vi "Delay.vi"(8 "error in (no error)":errorcluster, 9 "delay_value":u8=16 max=31 format="%1d", 10 "channel":u32, 11 "IP address":string="192.168.10.20") -> (0 "error out":errorcluster)   [LabVIEW 2017]
panel:
  in  "Read (TRUE)":bool
  out "Out":u8=16 format="%.0x"
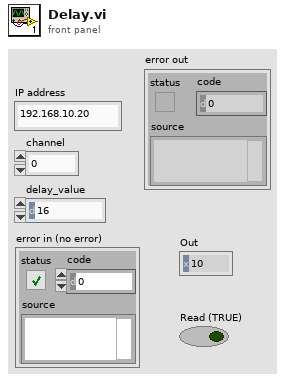
[diagram p1: front panel]
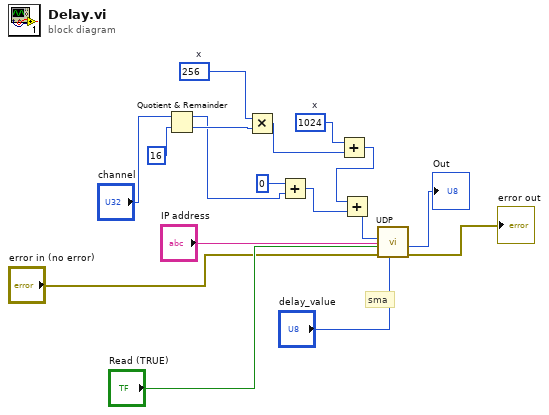
[diagram p0: block diagram]
diagram:
  w6 = u16 256  # x
  w4 = u16 1024  # x
  # "sma"
  n1 = Quotient & Remainder(x="channel", y=u32 16) -> (x-y*floor(x/y)=w1:u32, floor(x/y)=w5:u32)
  n2 = Multiply(x=w6, y=w5) -> (x*y=w3:u32)
  n3 = Add(x=u8 0, y=w1) -> (x+y=w11:u32)
  n4 = Add(x=w4, y=w3) -> (x+y=w2:u32)
  n5 = Add(x=w2, y=w11) -> (x+y=w15:u32)
  n6 = call "UDP.vi"("In"="delay_value", "error in (no error)"="error in (no error)", "Read (TRUE)"="Read (TRUE)", "Address"=w15, "IP address"="IP address") -> ("error out"=→"error out":errorcluster, "Out"=→"Out":u8)  [unwired: 4 in]
